vi "Get Trace Logs.vi"(8 "error in (no error)":errorcluster, 11 "Server in":refnum<class "Server.lvclass">) -> (0 "error out":errorcluster, 2 "Trace Logs":refnum<class "RequestTraceLog.lvclass">[](array[class]), 3 "Server out":refnum<class "Server.lvclass">)   [LabVIEW 2020, in "HTTP Server.lvlib" / "Server.lvclass"]
uses:
  Server.lvclass
  Server.lvclass/Server.ctl
  RequestTraceLog/RequestTraceLog.lvclass
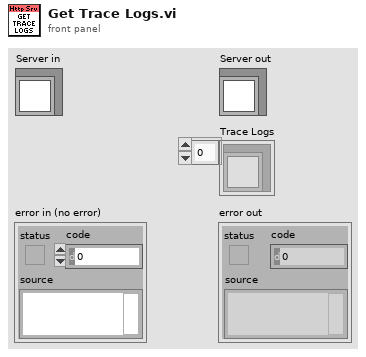
[diagram p1: front panel]
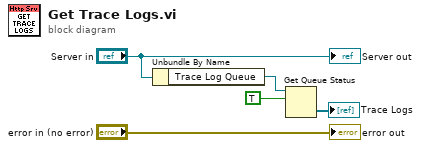
[diagram p0: block diagram]
diagram:
  n1 = Unbundle By Name("Server in") -> ("Trace Log Queue"=w3:refnum<queue>)
  n2 = Get Queue Status(queue=w3, return elements? (F)=TRUE) -> (elements=→"Trace Logs":refnum<class "RequestTraceLog.lvclass">[])  [unwired: 1 in, 7 out]
  "error out" <- "error in (no error)"
  "Server out" <- "Server in"
